vi "setAlignmentToDocument.vi"(8 "error in (no error)":errorcluster, 10 "Alignment":u16(ring) items=["LEFT"=1, "CENTER"=2, "RIGHT"=3, "BOTH"=4, "MEDIUM_KASHIDA"=5, "DISTRIBUTE"=6, "NUM_TAB"=7, "HIGH_KASHIDA"=8, "LOW_KASHIDA"=9, "THAI_DISTRIBUTE"=10], 11 "xwpfParagraph in":refnum<class "xwpfParagraph.lvclass">) -> (0 "error out":errorcluster, 3 "xwpfParagraph out":refnum<class "xwpfParagraph.lvclass">)   [LabVIEW 2017, in "Word_Specific.lvlib" / "xwpfParagraph.lvclass"]
uses:
  xwpfParagraph.lvclass
  xwpfParagraph.lvclass/xwpfParagraph.ctl
  C:/Users/Neo/Desktop/Dev_Tools_BR/LabVIEW_NPOI/lib/NPOI 2.1.1/NPOI.OOXML.dll
  lib/NPOI 2.1.1/NPOI.OOXML.dll
  Set Alignment.vi
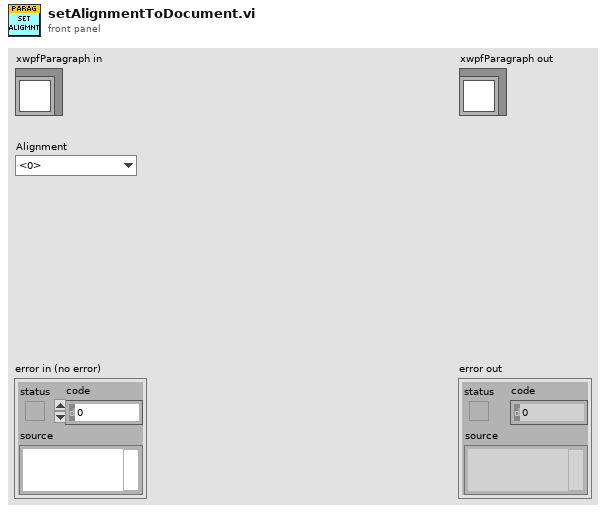
[diagram p1: front panel]
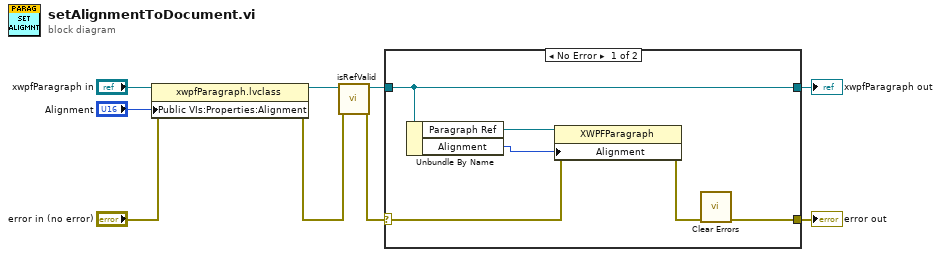
[diagram p0: block diagram]
diagram:
  n1 = property class="xwpfParagraph.lvclass"(reference="xwpfParagraph in", error in="error in (no error)", "Public VIs:Properties:Alignment"="Alignment") -> (reference out=w4:refnum<class "xwpfParagraph.lvclass">, error out=w2:errorcluster)
  n2 = call-dynamic "isRefValid.vi"("error in (no error)"=w2, "xwpfParagraph in"=w4) -> ("error out"=w1:errorcluster, "xwpfParagraph out"=w3:refnum<class "xwpfParagraph.lvclass">)  [unwired: 8 in]
  n3 = case shown="No Error" w1 {
    selector: w1 -> [w14 w17]
    tunnel: [w10 w17] -> w9
    tunnel: [w15 w16] -> w7
    tunnel: w3 -> [w15 w16]
    frame No Error {
      n4 = Unbundle By Name(w15) -> ("Paragraph Ref"=w11:refnum<k24>, "Alignment"=w12:u16)
      n5 = property class="XWPFParagraph"(reference=w11, error in=w14, "Alignment"=w12) -> (error out=w13:errorcluster)  [unwired: 1 out]
      n6 = call <vilib>:"Clear Errors.vi"("error in (no error)"=w13) -> ("error out"=w10:errorcluster)  [unwired: 5 in, 1 out]
    }
    frame Error {
    }
  }
  "error out" <- w9
  "xwpfParagraph out" <- w7
